vi "Write JSON Config.vi"(6 "Pretty Print?":bool, 8 "error in (no error)":errorcluster, 11 "AbsFunc_One Term_WFM_Numeric in":refnum<class "AbsFunc_One Term_WFM_Numeric.lvclass">) -> (0 "error out":errorcluster, 2 "JSON":string, 3 "AbsFunc_One Term_WFM_Numeric out":refnum<class "AbsFunc_One Term_WFM_Numeric.lvclass">)   [LabVIEW 2021, in "AbsFunc_One Term_WFM_Numeric.lvclass"]
uses:
  AbsFunc_One Term_WFM_Numeric.lvclass
  AbsFunc_One Term_WFM_Numeric.lvclass/AbsFunc_One Term_WFM_Numeric.ctl
  Abs_Types/Waveform/Abs_Waveform.lvclass
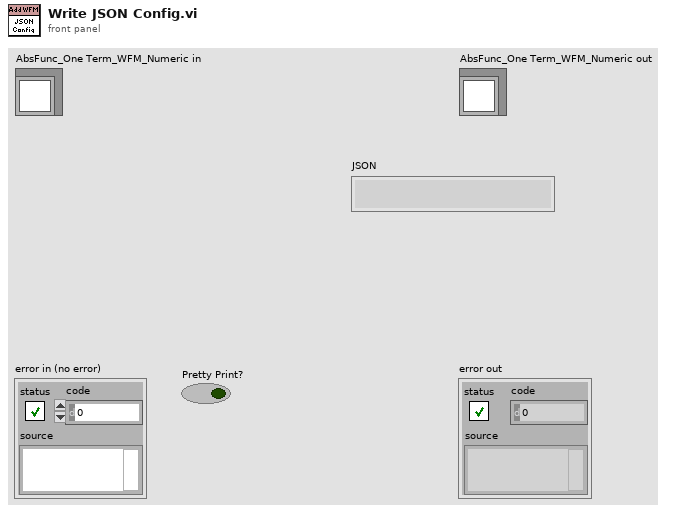
[diagram p1: front panel]
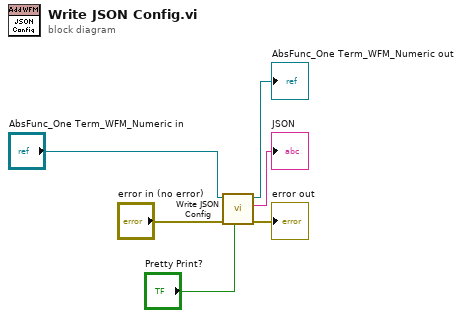
[diagram p0: block diagram]
diagram:
  n1 = call-parent "Write JSON Config.vi"("Pretty Print?"="Pretty Print?", "error in (no error)"="error in (no error)", "Abs_Type in"="AbsFunc_One Term_WFM_Numeric in") -> ("error out"=→"error out":errorcluster, "JSON"=→"JSON":string, "Abs_Type out"=→"AbsFunc_One Term_WFM_Numeric out":refnum<class "AbsFunc_One Term_WFM_Numeric.lvclass">)  [unwired: 6 in]
